vi "Boxcar Average.vi"(7 "reset":bool, 9 "sample length":i32=100, 10 "interleaved iq":i64[](array[numeric])) -> (1 "standard deviation":dbl format="%0.2f", 2 "trace":dbl format="%0.2f", 3 "mean":dbl format="%0.2f")   [LabVIEW 2017, in "Lock-In Amplifier Example Host.lvlib"]
uses:
  Lock-In Amplifier Example Host.lvlib
  <vilib>/Analysis/baseanly.llb/Mean (DBL).vi
  <vilib>/Analysis/NI_AALBase.lvlib
  <vilib>/ptbypt/NI_PtbyPt.lvlib
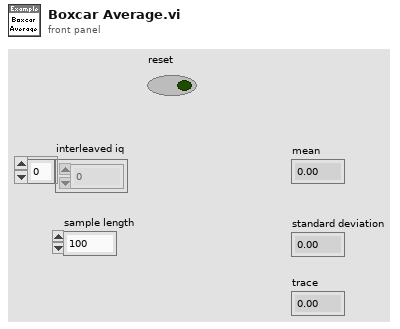
[diagram p1: front panel]
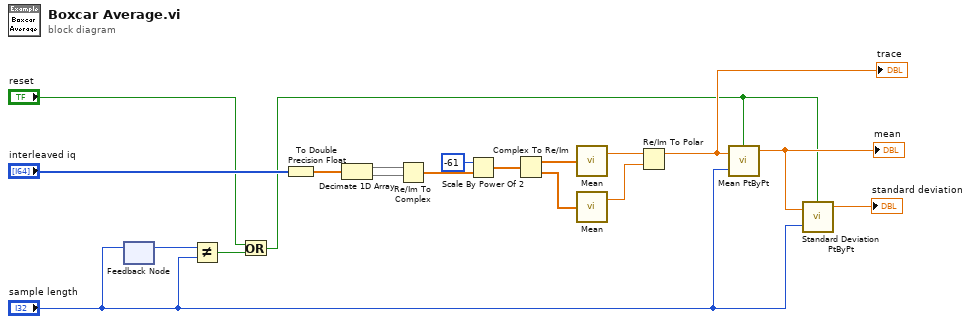
[diagram p0: block diagram]
diagram:
  n1 = feedback-in #1("sample length") -> ()
  n2 = feedback #1() -> (w3:i32)  [unwired: 1 in]
  n3 = Not Equal?(x=w3, y="sample length") -> (x != y?=w5:bool)
  n4 = Or(x="reset", y=w5) -> (x .or. y?=w2:bool)
  n5 = To Double Precision Float(number="interleaved iq") -> (double precision float=w7:dbl[])
  n6 = Decimate 1D Array(w7) -> (w9:dbl[], w8:dbl[])
  n7 = Re/Im To Complex(1:w8, 2:w9) -> (0:w6:cdb[])
  n8 = Scale By Power Of 2(n=i16 -61, x=w6) -> (x*2^n=w15:cdb[])
  n9 = Complex To Re/Im(x + iy=w15) -> (x=w14:dbl[], y=w10:dbl[])
  n10 = call-poly <vilib>:"Mean.vi"("X"=w14) -> ("mean"=w13:dbl)  [unwired: 1 out]
  n11 = call-poly <vilib>:"Mean.vi"("X"=w10) -> ("mean"=w11:dbl)  [unwired: 1 out]
  n12 = Re/Im To Polar(2:w11, 3:w13) -> (1:w12:dbl)  [unwired: 1 out]
  "trace" <- w12
  n13 = call <vilib>:"Mean PtByPt.vi"("x"=w12, "sample length"="sample length", "initialize"=w2) -> ("mean"=w17:dbl)  [unwired: 1 in, 1 out]
  "mean" <- w17
  n14 = call <vilib>:"Standard Deviation PtByPt.vi"("x"=w17, "sample length"="sample length", "initialize"=w2) -> ("standard deviation"=→"standard deviation":dbl)  [unwired: 2 out]
